vi "Read CurrName.vi"(8 "error in (no error)":errorcluster, 11 "HighscoreDialog in":refnum<class "HighscoreDialog.lvclass">) -> (0 "error out":errorcluster, 2 "CurrName":u8[](array[numeric]), 3 "HighscoreDialog out":refnum<class "HighscoreDialog.lvclass">)   [LabVIEW 2019, in "RT_Game.lvlib" / "HighscoreDialog.lvclass"]
uses:
  HighscoreDialog.lvclass
  HighscoreDialog.lvclass/HighscoreDialog.ctl
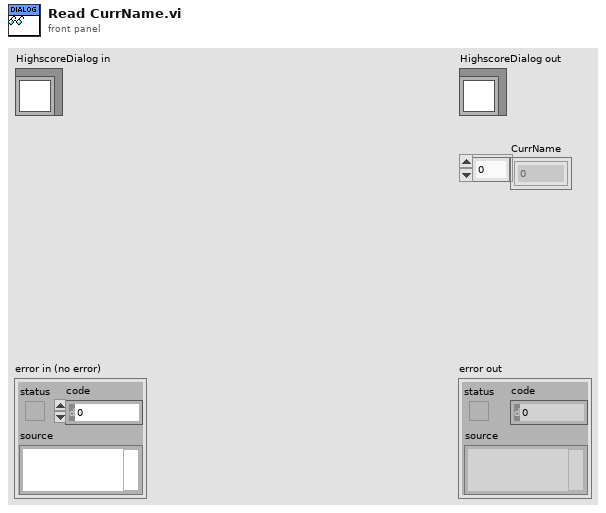
[diagram p1: front panel]
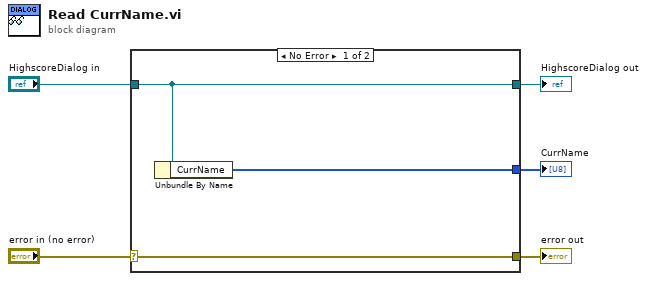
[diagram p0: block diagram]
diagram:
  n1 = case shown="No Error" "error in (no error)" {
    selector: "error in (no error)" -> [w8 w9]
    tunnel: [w8 w9] -> w4
    tunnel: [w7 w10] -> w2
    tunnel: "HighscoreDialog in" -> [w7 w10]
    tunnel: [w6 _] -> w1
    frame No Error {
      n2 = Unbundle By Name(w7) -> ("CurrName"=w6:u8[])
    }
    frame Error {
    }
  }
  "error out" <- w4
  "HighscoreDialog out" <- w2
  "CurrName" <- w1
